vi "Read HDF5.vi"(8 "error in (no error)":errorcluster, 11 "path":path) -> (0 "error out":errorcluster, 1 "Igor Commands":string, 2 "Notes":string, 3 "Data (Dictionary)":T1[](array[typedef]))   [LabVIEW 2020, in "Data.HDF5.lvclass"]
uses:
  Data.HDF5.lvclass
  <vilib>/addons/h5labview2/file/H5Fmode.ctl
  <vilib>/addons/h5labview2/base/H5Equery.vi
  <vilib>/addons/h5labview2/base/lib_path.vi
  <vilib>/UPVI/lvhdf5/dataset.llb/H5Dread.xnode
  Data/Typedefs/Dictionary--cluster.ctl
  Data/Data.lvclass
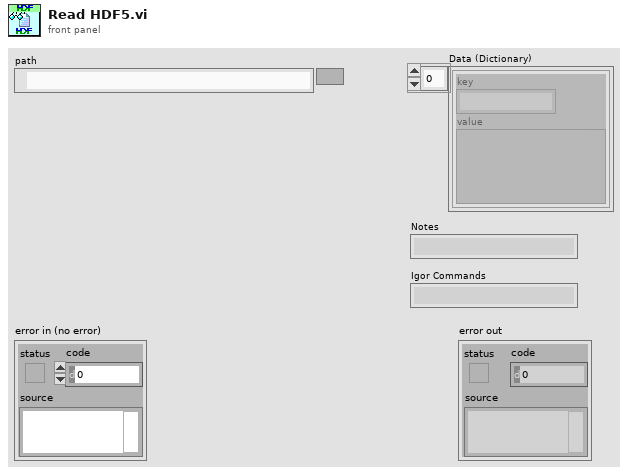
[diagram p1: front panel]
types:
  T1 = typedef "Data.lvclass/Dictionary--cluster.ctl" = cluster{"key":string, "value":variant}
  T2 = typedef "H5F.lvlib/H5Fmode.ctl" = enum16{"read-only", "read-write", "overwrite", "create new", "open or create"}
  T3 = typedef "hid_t.ctl" = i32
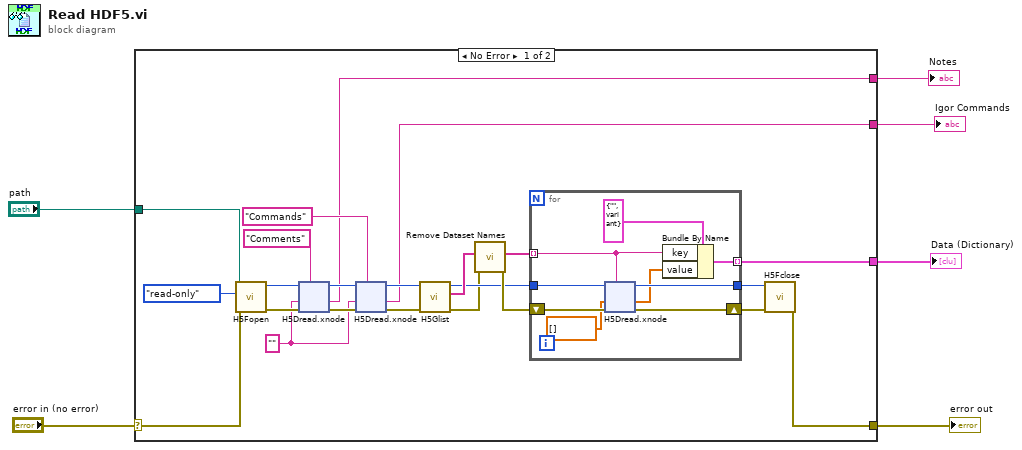
[diagram p0: block diagram]
diagram:
  n1 = case shown="No Error" "error in (no error)" {
    selector: "error in (no error)" -> [w11 w84]
    tunnel: [w23 w84] -> w5
    tunnel: "path" -> [w7 _]
    tunnel: [w10 _] -> w3
    tunnel: [w9 _] -> w2
    tunnel: [w8 _] -> w1
    frame No Error {
      w15 = "" ("attrib name")
      n2 = call <vilib>:"H5Fopen.vi"("error in (no error)"=w11, "mode (read-only)"=H5Fmode."read-only" ("mode"), "path"=w7) -> ("error out"=w28:errorcluster, "ref out"=w22:T3)  [unwired: 7 in]
      n3 = xnode "H5Dread.xnode"("dataset name (this)"="Comments" ("attrib name"), "error in (no error)"=w28, "default"=w15, "ref in"=w22) -> ("error out"=w26:errorcluster, "data"=w10:string, "ref out"=w25:i32)  [unwired: 2 in, 1 out]
      n4 = xnode "H5Dread.xnode"("dataset name (this)"="Commands" ("attrib name"), "error in (no error)"=w26, "default"=w15, "ref in"=w25) -> ("error out"=w13:errorcluster, "data"=w9:string, "ref out"=w21:i32)  [unwired: 2 in, 1 out]
      n5 = call <vilib>:"H5Glist.vi"("error in (no error)"=w13, "ref in"=w21) -> ("error out"=w12:errorcluster, "names"=w18:string[], "ref out"=w16:T3)  [unwired: 6 in, 1 out]
      n6 = call "Remove Dataset Names.vi"("error in (no error)"=w12, "Dataset Names"=w18) -> ("error out"=w17:errorcluster, "Name less Commands and Comments"=w14:string[])  [unwired: 8 in]
      n7 = for {
        shift-right: [w38] -> w20
        shift-left: w17 -> [w37]
        tunnel: w16 -> [w36]
        tunnel: [w35] -> w19
        tunnel: w14 -> [w31] mode=indexing
        tunnel: [w30] -> w8 mode=indexing
        n8 = xnode "H5Dread.xnode"("dataset name (this)"=w31, "error in (no error)"=w37, "default"=dbl[] [] ("array type (2D Dbl)"), "ref in"=w36) -> ("error out"=w38:errorcluster, "data"=w32:dbl[], "ref out"=w35:i32)  [unwired: 2 in, 1 out]
        n9 = Bundle By Name(cluster=T1 {"key"="", "value"=variant} ("key-value"), "key"=w31, "value"=w32) -> (w30:T1)
      }
      n10 = call <vilib>:"H5Fclose.vi"("error in (no error)"=w20, "ref"=w19) -> ("error out"=w23:errorcluster)  [unwired: 9 in]
    }
    frame Error {
    }
  }
  "error out" <- w5
  "Igor Commands" <- w2
  "Notes" <- w3
  "Data (Dictionary)" <- w1
